vi "ParseGISRepsonseString.vi"(8 "error in (no error)":errorcluster, 11 "Response In":string) -> (0 "error out":errorcluster, 1 "Status":string, 2 "ID":string, 3 "Category":string)   [LabVIEW 2022 SP3, in "GIS Printer.lvclass"]
uses:
  GIS Printer.lvclass
  <vilib>/regexp/Match Regular Expression.xnode
panel:
  # "A,[ID],P,P,1,C:\\Users\\labuser\\Desktop\\Scripts\\Patterns\\Head-Align\\PH1\\Indexed-dithered_1000wide_360x360dpi_rotated.bmp,1"
  # "I,[ID],RTP,1"
  # "C,[ID],0"
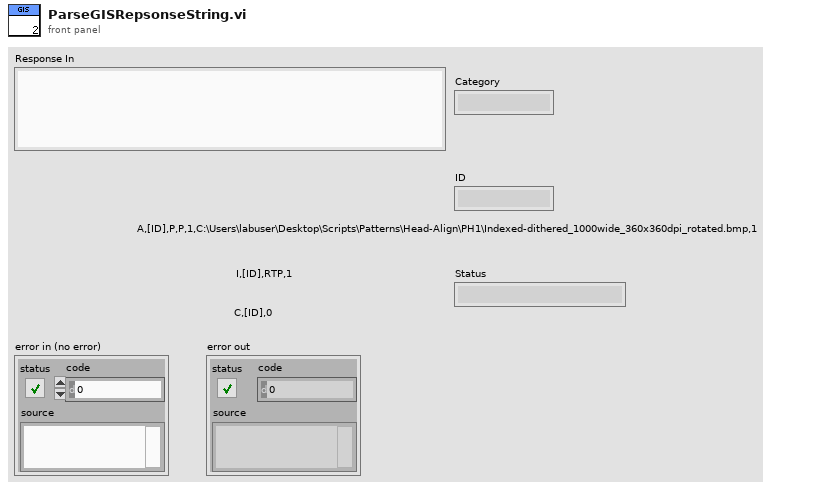
[diagram p1: front panel]
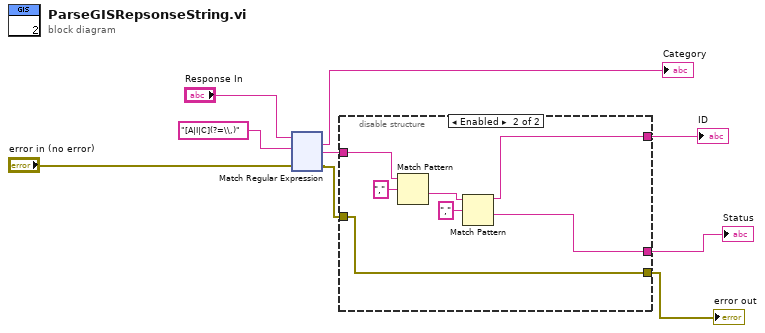
[diagram p0: block diagram]
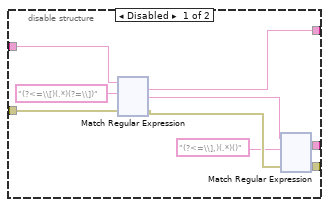
[diagram p2: hidden frame]
diagram:
  n1 = xnode "Match Regular Expression"("input string"="Response In", "regular expression"="[A|I|C](?=\\,)", "error in"="error in (no error)") -> ("whole match"=→"Category":string, "after match"=w2:string, "error out"=w7:errorcluster)  [unwired: 3 in, 2 out]
  n2 = disable-structure shown="Enabled" {
    disable-tunnel: [w18 w259] -> w8
    disable-tunnel: w7 -> [w16 w259]
    disable-tunnel: [w15 w253] -> w5
    disable-tunnel: [w12 w254] -> w4
    disable-tunnel: w2 -> [w10 w258]
    frame Disabled {
      n3 = xnode "Match Regular Expression"("input string"=w10, "regular expression"="(?<=\\[)(.*)(?=\\])", "error in"=w16) -> ("whole match"=w12:string, "after match"=w13:string, "error out"=w17:errorcluster)  [unwired: 3 in, 2 out]
      n4 = xnode "Match Regular Expression"("input string"=w13, "regular expression"="(?<=\\],)(.*)()", "error in"=w17) -> ("whole match"=w15:string, "error out"=w18:errorcluster)  [unwired: 3 in, 3 out]
    }
    frame Enabled {
      n5 = Match Pattern(string=w258, regular expression=",") -> (after substring=w255:string)  [unwired: 1 in, 3 out]
      n6 = Match Pattern(string=w255, regular expression=",") -> (before substring=w254:string, after substring=w253:string)  [unwired: 1 in, 2 out]
    }
  }
  "error out" <- w8
  "Status" <- w5
  "ID" <- w4
